vi "Update inventory.vi"(9 "Producto":string[](array[string]), 10 "Products":enum16{"Bakery", "Coffee"}(ring), 11 "Message Enqueuer in":refnum<class "Message Enqueuer.lvclass">) -> ()   [LabVIEW 2019, in "UI Actor.lvlib" / "UI Actor.lvclass"]
uses:
  UI Actor.lvclass
  <vilib>/ActorFramework/Message Enqueuer/Message Enqueuer.lvclass
  <vilib>/ActorFramework/Message Enqueuer/Message Enqueuer.lvclass/Message Enqueuer.ctl
  <vilib>/ActorFramework/Message Enqueuer/Enqueue.vi
  Bakery Actor Messages/Init Msg/Init Msg.lvclass
  C:/Program Files/National Instruments/LabVIEW 2019/vi.lib/ActorFramework/Message/Message.lvclass
  Coffee Actor Messages/init Msg/init Msg.lvclass
  <vilib>/Utility/config.llb/Write Key (String).vi
  <vilib>/ActorFramework/Message Priority Queue/Priority Enqueue.vi
  <vilib>/Utility/config.llb/NI_LVConfig.lvlib
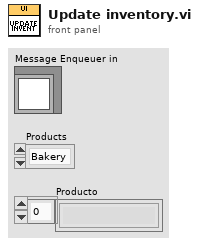
[diagram p1: front panel]
types:
  T1 = typedef "NI_LVConfig.lvlib/Config Data RefNum.ctl" = refnum<k1>
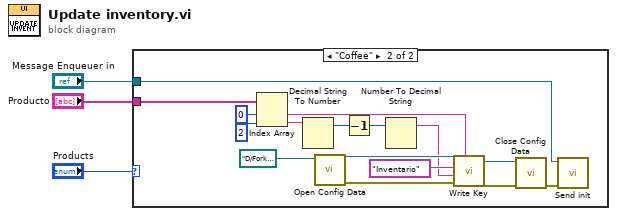
[diagram p0: block diagram]
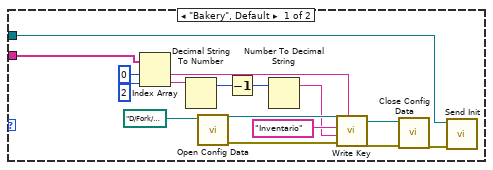
[diagram p2: hidden frame]
diagram:
  n1 = case shown="\"Coffee\"" "Products" {
    tunnel: "Producto" -> [w6 w23]
    tunnel: "Message Enqueuer in" -> [w5 w20]
    frame "Bakery", Default {
      n2 = Index Array(array=w6, index #1=0 ("index"), index #2=2 ("index")) -> (element #1=w14:string, element #2=w11:string)
      n3 = Decimal String To Number(string=w11) -> (number=w10:i32)  [unwired: 2 in, 1 out]
      n4 = call <vilib>:"Open Config Data.vi"("configuration file path"=path "D:/Fork/AF MaqExp-2Parcial/Bakery Actor.ini") -> ("error out"=w16:errorcluster, "refnum"=w17:T1)  [unwired: 8 in, 1 out]
      n5 = Decrement(x=w10) -> (x-1=w9:i32)
      n6 = Number To Decimal String(number=w9) -> (decimal integer string=w8:string)  [unwired: 1 in]
      n7 = call-poly <vilib>:"Write Key.vi"("section"=w14, "error in (no error)"=w16, "value"=w8, "key"="Inventario" ("section"), "refnum"=w17) -> ("error out"=w18:errorcluster, "refnum out"=w19:T1)  [unwired: 4 in, 1 out]
      n8 = call <vilib>:"Close Config Data.vi"("error in (no error)"=w18, "refnum"=w19) -> ("error out"=w4:errorcluster)  [unwired: 8 in, 1 out]
      n9 = call "Send Init.vi"("error in (no error)"=w4, "Message Enqueuer"=w5) -> ()  [unwired: 8 in, 2 out]
    }
    frame "Coffee" {
      n10 = Index Array(array=w23, index #1=0 ("index"), index #2=2 ("index")) -> (element #1=w30:string, element #2=w27:string)
      n11 = Decimal String To Number(string=w27) -> (number=w26:i32)  [unwired: 2 in, 1 out]
      n12 = call <vilib>:"Open Config Data.vi"("configuration file path"=path "D:/Fork/AF MaqExp-2Parcial/Coffee Actor.ini") -> ("error out"=w32:errorcluster, "refnum"=w33:T1)  [unwired: 8 in, 1 out]
      n13 = Decrement(x=w26) -> (x-1=w25:i32)
      n14 = Number To Decimal String(number=w25) -> (decimal integer string=w24:string)  [unwired: 1 in]
      n15 = call-poly <vilib>:"Write Key.vi"("section"=w30, "error in (no error)"=w32, "value"=w24, "key"="Inventario" ("section"), "refnum"=w33) -> ("error out"=w34:errorcluster, "refnum out"=w35:T1)  [unwired: 4 in, 1 out]
      n16 = call <vilib>:"Close Config Data.vi"("error in (no error)"=w34, "refnum"=w35) -> ("error out"=w21:errorcluster)  [unwired: 8 in, 1 out]
      n17 = call "Send init.vi"("error in (no error)"=w21, "Message Enqueuer"=w20) -> ()  [unwired: 8 in, 2 out]
    }
  }
